vi "Dictionary Test - 009.vi"(8 "error in (no error)":errorcluster) -> (0 "error out":errorcluster, 2 "pass":bool)   [LabVIEW 2009]
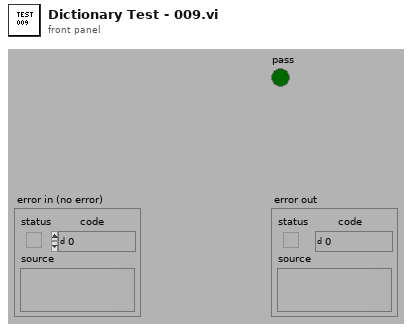
[diagram p1: front panel]
types:
  T1 = typedef "Dictionary Object RefNum.ctl" = refnum<k1>
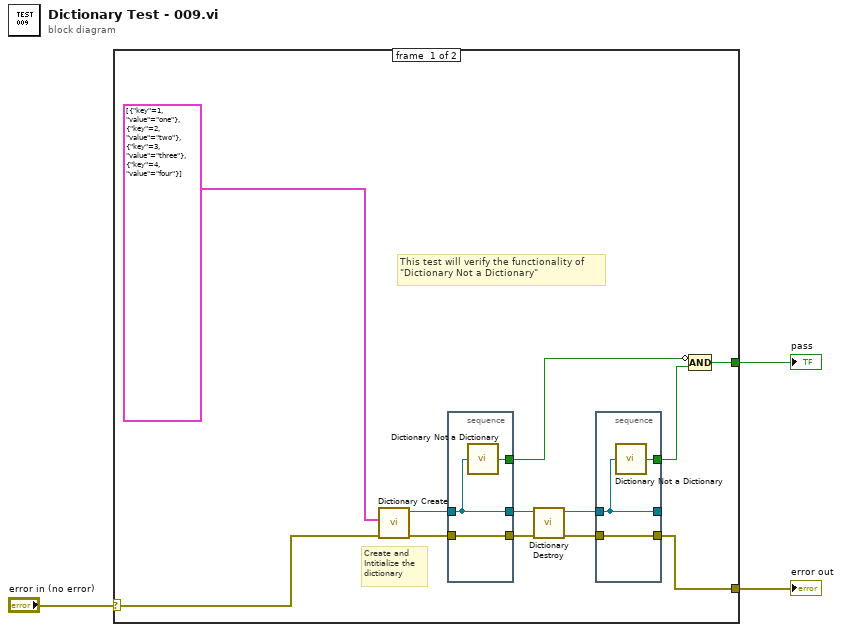
[diagram p0: block diagram]
diagram:
  n1 = case shown="No Error" "error in (no error)" {
    selector: "error in (no error)" -> [w14 w21]
    tunnel: [w4 w21] -> w1
    tunnel: [w13 _] -> w3
    frame #0 {
      # "Create and Intitialize the dictionary"
      # "This test will verify the functionality of \n\"Dictionary Not a Dictionary\""
      n2 = call "Dictionary Create.vi"("error in (no error)"=w14, "initial dictionary (empty)"=cluster{"key":i32, "value":string}[] [{"key"=1, "value"="one"}, {"key"=2, "value"="two"}, {"key"=3, "value"="three"}, {"key"=4, "value"="four"}] ("dictionary with updates")) -> ("error out"=w10:errorcluster, "dictionary out"=w12:T1)  [unwired: 8 in]
      n3 = stacked-sequence {
        tunnel: w12 -> [w20]
        tunnel: w10 -> [w19]
        tunnel: [w19] -> w9
        tunnel: [w18] -> w6
        tunnel: [w20] -> w8
        frame #0 {
          n4 = call "Dictionary Not a Dictionary.vi"("dictionary"=w20) -> ("not a dictionary?"=w18:bool)
        }
      }
      n5 = call "Dictionary Destroy.vi"("error in (no error)"=w9, "dictionary"=w8) -> ("error out"=w7:errorcluster)  [unwired: 9 in]
      n6 = stacked-sequence {
        tunnel: w8 -> [w17]
        tunnel: w7 -> [w16]
        tunnel: [w16] -> w4
        tunnel: [w15] -> w5
        tunnel: [w17] -> _
        frame #0 {
          n7 = call "Dictionary Not a Dictionary.vi"("dictionary"=w17) -> ("not a dictionary?"=w15:bool)
        }
      }
      n8 = Compound Arithmetic op=AND(invert w6, w5) -> (w13:bool)
    }
    frame #1 {
    }
  }
  "pass" <- w3
  "error out" <- w1
